vi "APC_9049_NI9222conf.vi"() -> (0 "Min V out":dbl[](array[numeric])=[-10.0, -10.0, -10.0, -10.0, -10.0, -10.0, -10.0, -10.0, -10.0], 1 "Max V out":dbl[](array[numeric])=[10.0, 10.0, 10.0, 10.0, 10.0, 10.0, 10.0, 10.0, 10.0], 2 "scaled units out":string[](array[string])=["bar", "bar", "bar", "bar", "bar", "bar", "bar", "bar", "bar"], 3 "Y-Intercept out":dbl[](array[numeric])=[0.0, 5.0, 10.0, 15.0, 0.0, 0.0, 0.0, 0.0, 0.0] format="%.2g", 4 "Slope out":dbl[](array[numeric])=[1.0, 1.0, 1.0, 100.0, 1.0, 1.0, 1.0, 1.0, 1.0] format="%.2g", 5 "channels name out":string[](array[string])=["Pcyl1", "Pcyl2", "Pcyl3", "Pcyl4", "Pcyl5", "Pcyl6", "Ppre", "Psyst", "Pexh"])   [LabVIEW 2020]
panel:
  in  "Min V":dbl[](array[numeric])=[-10.0, -10.0, -10.0, -10.0, -10.0, -10.0, -10.0, -10.0, -10.0]
  in  "Max V":dbl[](array[numeric])=[10.0, 10.0, 10.0, 10.0, 10.0, 10.0, 10.0, 10.0, 10.0]
  in  "scaled units":string[](array[string])=["bar", "bar", "bar", "bar", "bar", "bar", "bar", "bar", "bar"]
  in  "Y-Intercept":dbl[](array[numeric])=[0.0, 5.0, 10.0, 15.0, 0.0, 0.0, 0.0, 0.0, 0.0] format="%.2g"
  in  "Slope":dbl[](array[numeric])=[1.0, 1.0, 1.0, 100.0, 1.0, 1.0, 1.0, 1.0, 1.0] format="%.2g"
  in  "channels name":string[](array[string])=["Pcyl1", "Pcyl2", "Pcyl3", "Pcyl4", "Pcyl5", "Pcyl6", "Ppre", "Psyst", "Pexh"]
  # "NI9222"
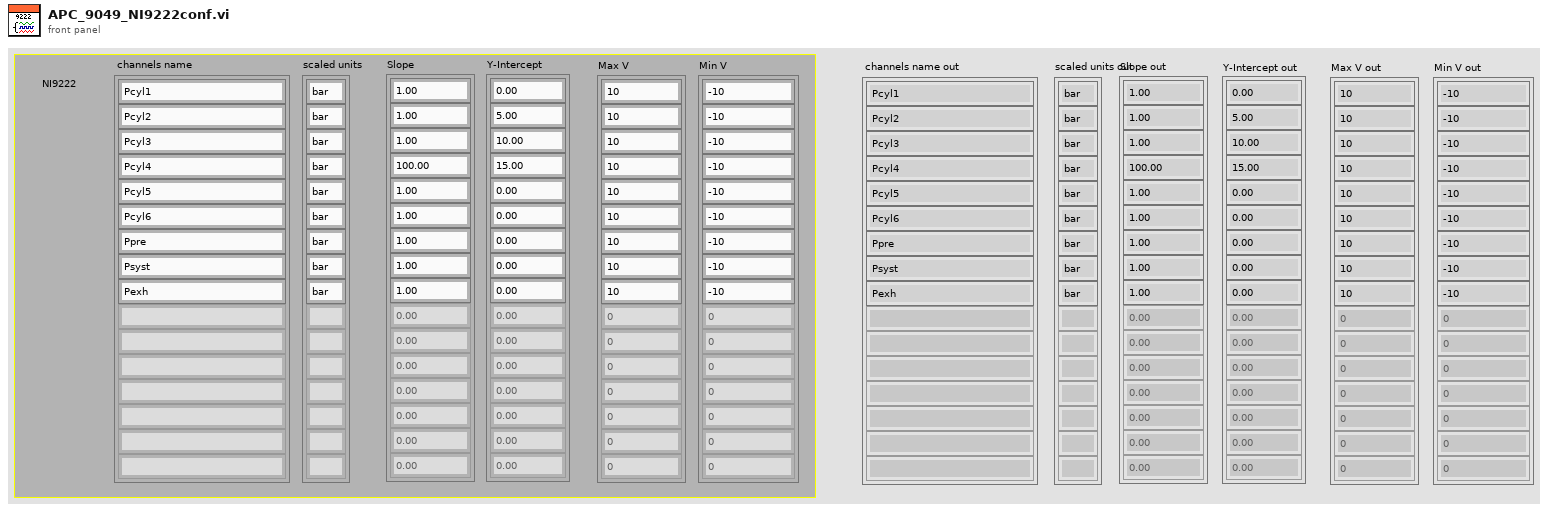
[diagram p1: front panel]
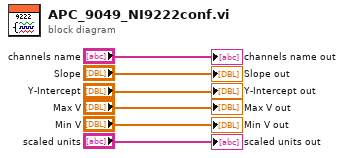
[diagram p0: block diagram]
diagram:
  "channels name out" <- "channels name"
  "Slope out" <- "Slope"
  "Y-Intercept out" <- "Y-Intercept"
  "Max V out" <- "Max V"
  "Min V out" <- "Min V"
  "scaled units out" <- "scaled units"
